vi "Results to Waveforms (array of waveforms).vi"(1 "data type":waveform(dbl)[](array[waveform]), 7 "result references":T1[](array[typedef]), 11 "error in (no error)":errorcluster) -> (6 "signals out":waveform(dbl)[](array[waveform]), 8 "result references out":T1[](array[typedef]), 15 "error out":errorcluster)   [LabVIEW 2020, in "NI_DataFinder.lvlib"]
doc: "Extracts the signals from the results of a DataFinder search."
uses:
  <vilib>/DataFinder/NI_DataFinder.lvlib
  <vilib>/userdefined/DFSearchResult.ctl
  <vilib>/userdefined/NI_DataFinder Controls.lvlib
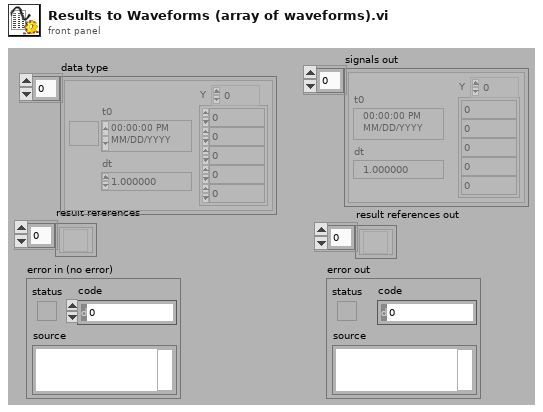
[diagram p1: front panel]
types:
  T1 = typedef "NI_DataFinder Controls.lvlib/DFSearchResult.ctl" = refnum<k20>
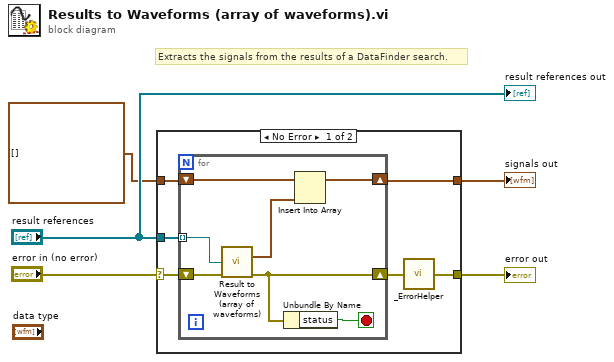
[diagram p0: block diagram]
diagram:
  # "Extracts the signals from the results of a DataFinder search."
  n1 = case shown="No Error" "error in (no error)" {
    selector: "error in (no error)" -> [w10 w19]
    tunnel: "result references" -> [w11 _]
    tunnel: waveform(dbl)[] [] ("Signals out") -> [w8 w20]
    tunnel: [w9 w20] -> w2
    tunnel: [w6 w19] -> w1
    frame No Error {
      n2 = for {
        tunnel: w11 -> [w18] mode=indexing
        shift-right: [w13] -> w7
        shift-left: w10 -> [w17]
        shift-right: [w16] -> w9
        shift-left: w8 -> [w15]
        stop <- w14 stop-if-true
        n3 = call <vilib>:"Result to Waveforms (array of waveforms).vi"("result reference"=w18, "error in"=w17) -> ("signals out"=w12:waveform(dbl)[], "error out"=w13:errorcluster)  [unwired: 12 out]
        n4 = Unbundle By Name(w13) -> ("status"=w14:bool)
        n5 = Insert Into Array(array=w15, new element=w12) -> (w16:waveform(dbl)[])  [unwired: 1 in]
      }
      n6 = call <vilib>:"_ErrorHelper.vi"("error IO"=w7) -> ("error out"=w6:errorcluster)
    }
    frame Error {
    }
  }
  "error out" <- w1
  "signals out" <- w2
  "result references out" <- "result references"
